vi "Test SuiteDestructionError.vi"(8 "error in (no error)":errorcluster) -> (0 "error out":errorcluster)   [LabVIEW 2020]
uses:
  classes/Test Suite/Test Suite.lvclass
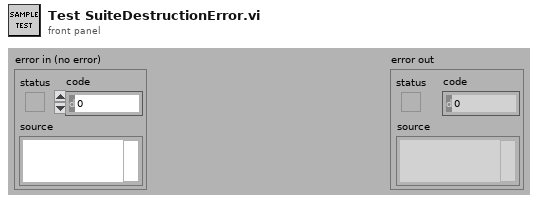
[diagram p1: front panel]
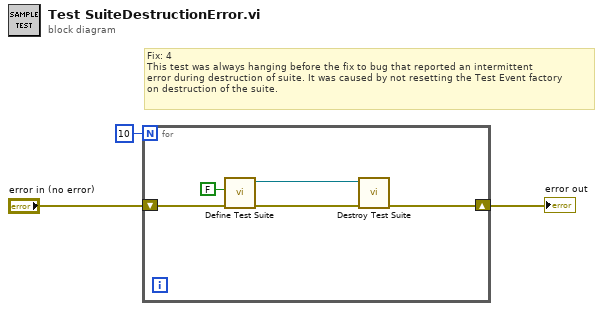
[diagram p0: block diagram]
diagram:
  # "Fix: 4\nThis test was always hanging before the fix to bug that reported an intermittent\nerror during destruction of suite. It was caused by not resetting the Test Event factory\non destruction of the suite."
  n1 = for {
    N: 10 -> [_]
    shift-right: [w6] -> w1
    shift-left: "error in (no error)" -> [w8]
    n2 = call "Define Test Suite.vi"("error in (no error)"=w8, "Interactive"=FALSE) -> ("error out"=w7:errorcluster, "Test Suite"=w4:refnum<class "Test Suite.lvclass">)  [unwired: 7 in, 1 out]
    n3 = call-dynamic "Destroy Test Suite.vi"("error in (no error)"=w7, "Test Suite in"=w4) -> ("error out"=w6:errorcluster)  [unwired: 8 in, 1 out]
  }
  "error out" <- w1
